vi "Construct.vi"(8 "error in (no error)":errorcluster, 11 "CRuleList in":refnum<class "CRuleList.lvclass">) -> (0 "error out":errorcluster, 3 "CRuleList out":refnum<class "CRuleList.lvclass">)   [LabVIEW 2020, in "DependencyInspection.lvlib" / "CRuleList.lvclass"]
uses:
  CRuleList.lvclass
  LabVIEWObjectInterfaces/IDependencyItemRule/IDependencyItemRule.lvclass
  RuleList.ctl
  E:/Repos/LVDependencyInspector/src/LabVIEWObjectInterfaces/IDependencyItemRule/IDependencyItemRule.lvclass
  E:/Repos/LVDependencyInspector/src/LabVIEWObjectInterfaces/ILabVIEWItem/ILabVIEWItem.lvclass
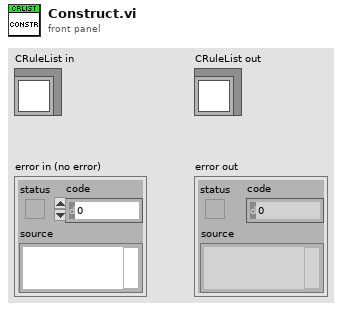
[diagram p1: front panel]
types:
  T1 = typedef "DependencyInspection.lvlib/CRuleList.lvclass/RuleList.ctl" = map{string, refnum<class "IDependencyItemRule.lvclass">}
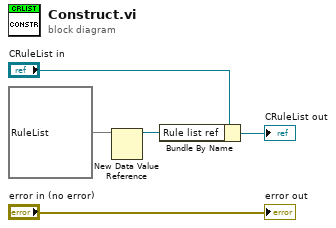
[diagram p0: block diagram]
diagram:
  n1 = New Data Value Reference(data value=T1 {} ("Rule List")) -> (data value reference=w1:refnum<data-value>)  [unwired: 1 in, 1 out]
  n2 = Bundle By Name(cluster="CRuleList in", "Rule list ref"=w1) -> (→"CRuleList out":refnum<class "CRuleList.lvclass">)
  "error out" <- "error in (no error)"
